vi "Read logs.vi"() -> ()   [LabVIEW 2020]
panel:
  in  "Choose file":bool
  out "error out":errorcluster
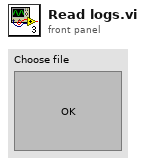
[diagram p1: front panel]
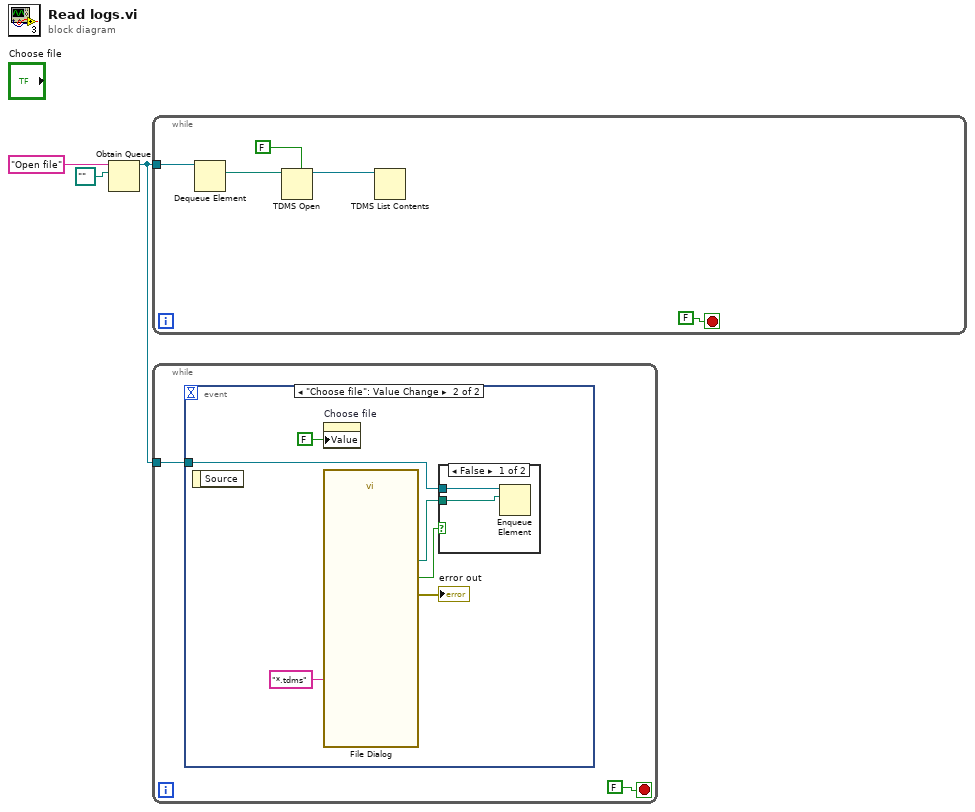
[diagram p0: block diagram]
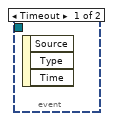
[diagram p2: hidden frame]
diagram:
  n1 = Obtain Queue(name (unnamed)="Open file", element data type=path "") -> (queue out=w1:refnum<queue>)  [unwired: 3 in, 2 out]
  n2 = while {
    tunnel: w1 -> [w7]
    stop <- FALSE stop-if-true
    n3 = Dequeue Element(queue=w7) -> (element=w6:path)  [unwired: 2 in, 3 out]
    n4 = TDMS Open(5:FALSE ("create index file? (T)"), 11:w6) -> (3:w4:refnum<k34>)  [unwired: 5 in, 1 out]
    n5 = TDMS List Contents(7:w4) -> ()  [unwired: 2 in, 4 out]
  }
  n6 = while {
    tunnel: w1 -> [w9]
    stop <- FALSE stop-if-true
    n7 = event shown="[1] \"Choose file\": Value Change" {
      selector: _ -> [_ _]
      dyn-events: _ -> [_ _]
      timeout: _ -> [_ _]
      tunnel: w9 -> [_ w11]
      event Timeout {
        n8 = event-data() -> ()  [unwired: 1 in, 3 out]
      }
      event "Choose file": Value Change {
        n9 = event-data() -> ()  [unwired: 1 in, 1 out]
        n10 = property on="Choose file" class="Bool (strict)"("Value"=FALSE ("Choose file")) -> ()  [unwired: 2 in, 2 out]
        n11 = call "File Dialog"("pattern (all files)"="*.tdms") -> ("selected path"=w12:path, "cancelled"=w13:bool, "error out"=→"error out":errorcluster)  [unwired: 11 in, 1 out]
        n12 = case shown="False" w13 {
          tunnel: w12 -> [w17 _]
          tunnel: w11 -> [w18 _]
          frame False {
            n13 = Enqueue Element(queue=w18, element=w17) -> ()  [unwired: 2 in, 3 out]
          }
          frame True {
          }
        }
      }
    }
  }
